vi "Get All Minor Frames.vi"(8 "error in (no error)":errorcluster, 11 "Major Frame in":refnum<class "Major Frame.lvclass">) -> (0 "error out":errorcluster, 1 "Minor Frames":refnum<class "Minor Frame.lvclass">[](array[class]), 2 "Minor Frame IDs":string[](array[string]), 3 "Major Frame out":refnum<class "Major Frame.lvclass">)   [LabVIEW 2020, in "BCI-1553 API.lvlib" / "Major Frame.lvclass"]
doc: "Retrieves a list of all the Minor Frames available to this Major Frame."
uses:
  Major Frame.lvclass
  Minor Frame/Minor Frame.lvclass
  Major Frame.lvclass/Major Frame.ctl
  Dependencies/Registry/Registry.lvclass/Registry.ctl
  Dependencies/Registry/Registry.lvclass
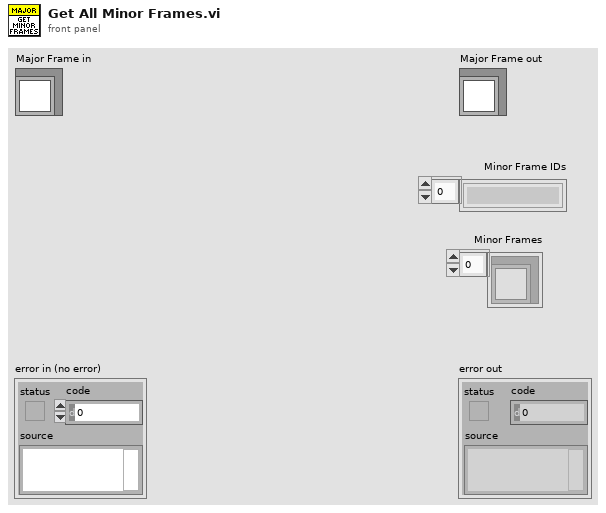
[diagram p1: front panel]
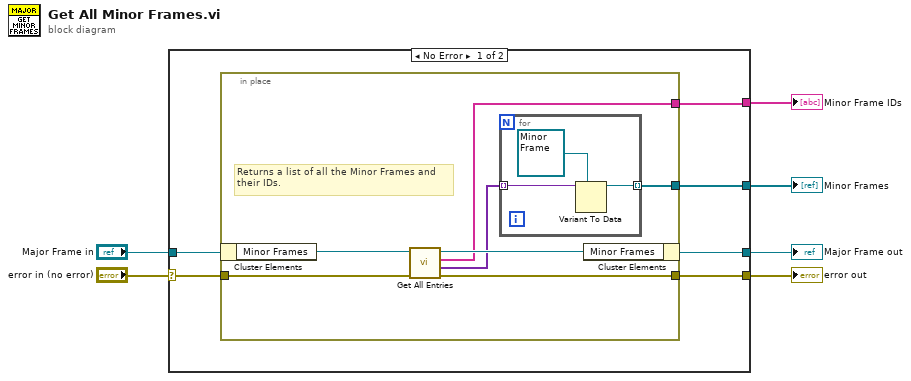
[diagram p0: block diagram]
diagram:
  n1 = case shown="No Error" "error in (no error)" {
    selector: "error in (no error)" -> [w9 w23]
    tunnel: [w10 w23] -> w5
    tunnel: [w11 w22] -> w3
    tunnel: "Major Frame in" -> [w12 w22]
    tunnel: [w8 _] -> w2
    tunnel: [w7 _] -> w1
    frame No Error {
      n2 = in-place {
        in-place-border: [w16] -> w10
        in-place-border: w9 -> [w17]
        in-place-border: [w15] -> w7
        in-place-border: [w13] -> w8
        # "Returns a list of all the Minor Frames and\ntheir IDs."
        n3 = in-place-cluster #1(w12) -> ("Minor Frames"=w18:refnum<class "Registry.lvclass">)
        n4 = call "Get All Entries.vi"("error in (no error)"=w17, "Registry in"=w18) -> ("error out"=w16:errorcluster, "Values"=w14:variant[], "Keys"=w15:string[])  [unwired: 7 in]
        n5 = for {
          tunnel: w14 -> [w21] mode=indexing
          tunnel: [w19] -> w13 mode=indexing
          n6 = Variant To Data(type=refnum<class "Minor Frame.lvclass"> refnum ("SLSC 1553 API.lvlib:Minor Frame.lvclass"), Variant=w21) -> (data=w19:refnum<class "Minor Frame.lvclass">)  [unwired: 1 in, 1 out]
        }
        n7 = in-place-cluster #1("Minor Frames"=w18) -> (w11:refnum<class "Major Frame.lvclass">)
      }
    }
    frame Error {
    }
  }
  "error out" <- w5
  "Major Frame out" <- w3
  "Minor Frames" <- w2
  "Minor Frame IDs" <- w1
